vi "Initiate Front Panel Data.vi"(8 "error in":errorcluster, 11 "Water Tunnel Results in":refnum<class "Water Tunnel Results.lvclass">) -> (0 "error out":errorcluster, 3 "Water Tunnel Results out":refnum<class "Water Tunnel Results.lvclass">)   [LabVIEW 2019, in "Results.lvlib" / "Water Tunnel Results.lvclass"]
uses:
  Water Tunnel Results.lvclass
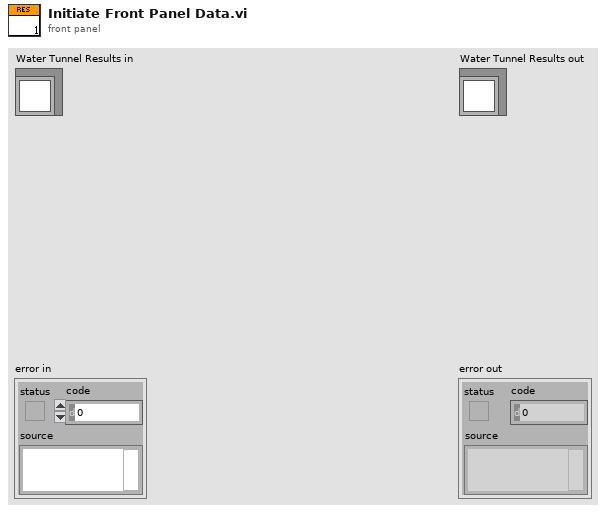
[diagram p1: front panel]
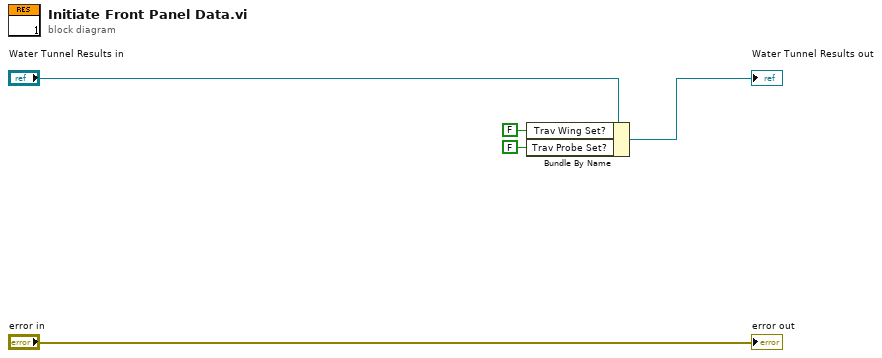
[diagram p0: block diagram]
diagram:
  n1 = Bundle By Name(cluster="Water Tunnel Results in", "Trav Wing Set?"=FALSE, "Trav Probe Set?"=FALSE) -> (→"Water Tunnel Results out":refnum<class "Water Tunnel Results.lvclass">)
  "error out" <- "error in"
